vi "Send Log Data DBL.vi"(6 "Time Stamp":timestamp format="%<%x %.3X>T", 7 "Message Priority (Normal)":T1=enum."Normal", 8 "error in (no error)":errorcluster, 9 "DBL":dbl, 10 "Ident":string, 11 "Message Enqueuer":refnum<class "Message Enqueuer.lvclass">) -> (0 "error out":errorcluster, 3 "Message Enqueuer out":refnum<class "Message Enqueuer.lvclass">)   [LabVIEW 2023, in "ISeries Actor.lvlib" / "Log Data DBL Msg.lvclass"]
doc: "This VI sends the message to an actor."
uses:
  Log Data DBL Msg.lvclass
  Log Data DBL Msg.lvclass/Log Data DBL Msg.ctl
  <vilib>/ActorFramework/Message Enqueuer/Message Enqueuer.lvclass
  C:/Program Files/National Instruments/LabVIEW 2023/vi.lib/ActorFramework/Message/Message.lvclass
  D:/git/HAL/HAL GOOP4/Series/ISeries Actor/ISeries Actor Messages/Log Data DBL Msg/Log Data DBL Msg.lvclass
  <vilib>/ActorFramework/Message Enqueuer/Message Priority.ctl
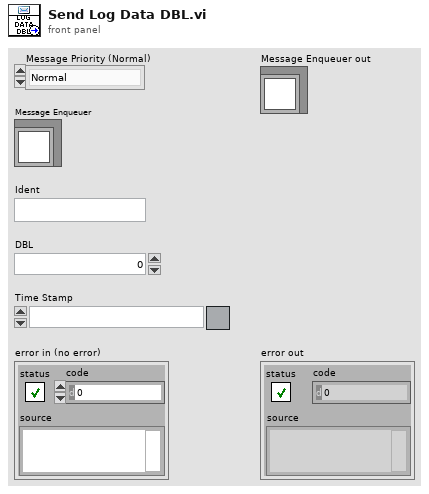
[diagram p1: front panel]
types:
  T1 = typedef "Actor Framework.lvlib/Message Enqueuer.lvclass/Message Priority.ctl" = enum16{"Low", "Normal", "High"}
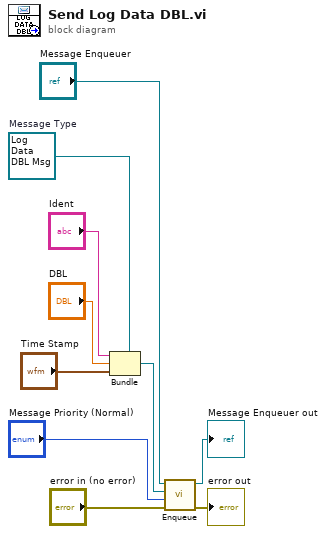
[diagram p0: block diagram]
diagram:
  w7 = refnum<class "Log Data DBL Msg.lvclass"> refnum  # Message Type
  n1 = Bundle(cluster=w7, "Ident", "DBL", "Time Stamp") -> (w6:refnum<class "Log Data DBL Msg.lvclass">)
  n2 = call <vilib>:"Enqueue.vi"("error in (no error)"="error in (no error)", "Message Priority (Normal)"="Message Priority (Normal)", "Message"=w6, "Message Enqueuer in"="Message Enqueuer") -> ("error out"=→"error out":errorcluster, "Message Enqueuer in"=→"Message Enqueuer out":refnum<class "Message Enqueuer.lvclass">)  [unwired: 6 in]
